vi "Console.vi"() -> ()   [LabVIEW 2017]
uses:
  Print Options.ctl
panel:
  out "Console Out":string
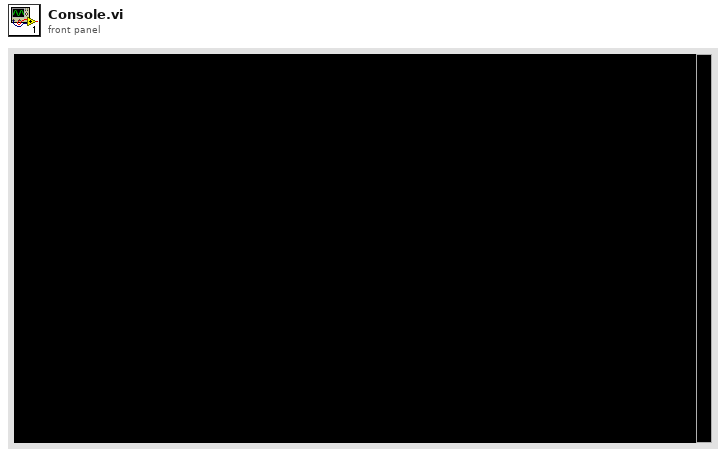
[diagram p1: front panel]
types:
  T1 = typedef "Print Options.ctl" = enum16{"Create", "Get Reference", "Print", "Print Header", "Close"}
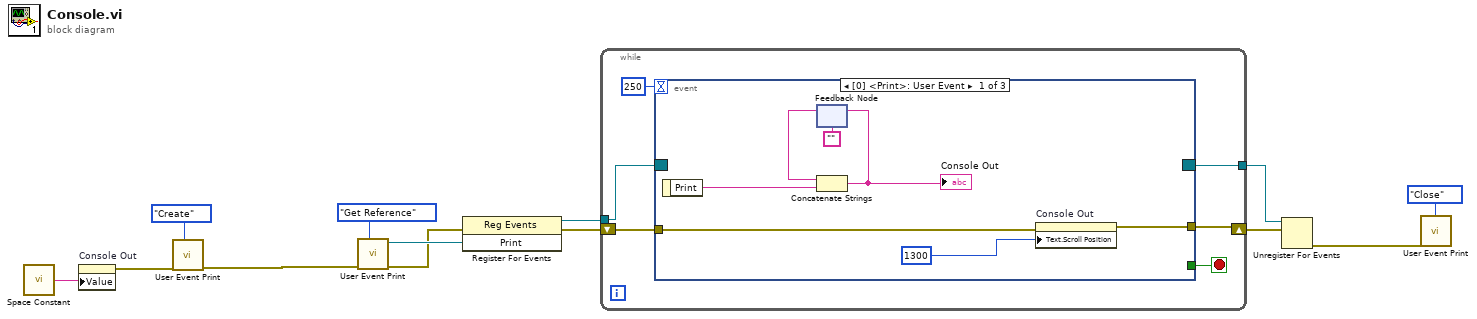
[diagram p0: block diagram]
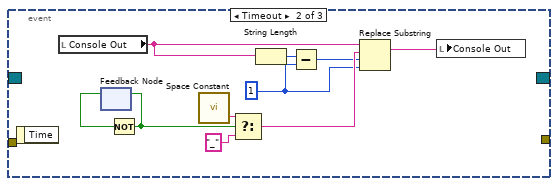
[diagram p2: hidden frame]
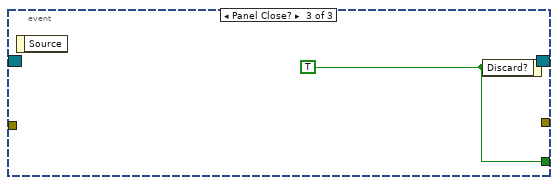
[diagram p3: hidden frame]
diagram:
  n1 = call <vilib>:"Space Constant.vi"() -> ("String"=w4:string)
  n2 = property on="Console Out" class="Str"("Value"=w4) -> (error out=w5:errorcluster)  [unwired: 2 in, 1 out]
  n3 = call "User Event Print.vi"("Options"=Print_Options."Create", "error in (no error)"=w5) -> ("error out"=w7:errorcluster)  [unwired: 8 in, 1 out]
  n4 = call "User Event Print.vi"("Options"=Print_Options."Get Reference", "error in (no error)"=w7) -> ("error out"=w3:errorcluster, "Print"=w6:refnum<user-event>)  [unwired: 8 in]
  n5 = register-events(error in=w3, w6) -> (reference out=w12:refnum<event-registration>, error out=w2:errorcluster)  [unwired: 1 in]
  n6 = while {
    tunnel: w12 -> [w18]
    tunnel: [w17] -> w13
    shift-right: [w14] -> w1
    shift-left: w2 -> [w15]
    stop <- w19 stop-if-true
    n7 = event shown="[0] <Print>: User Event" {
      selector: w18 -> [_ _ _]
      dyn-events: [_ _ _] -> w17
      timeout: 250 -> [_ _ _]
      tunnel: [_ _ w37] -> w19
      tunnel: w15 -> [w21 _ _]
      tunnel: [w20 _ _] -> w14
      event User Event {
        n8 = event-data() -> ("Print"=w26:string)  [unwired: 1 in]
        n9 = feedback #1("") -> (w25:string)
        n10 = Concatenate Strings(w25, w26) -> (w23:string)
        "Console Out" <- w23
        n11 = feedback-in #1(w23) -> ()
        n12 = property on="Console Out" class="Str"(error in=w21, "Text.Scroll Position"=u32 1300) -> (error out=w20:errorcluster)  [unwired: 1 in, 1 out]
      }
      event Timeout {
        w29 = 1 ("length (len. of substring)")
        n13 = event-data() -> ()  [unwired: 1 in, 1 out]
        n14 = local read "Console Out"() -> (w34:string)
        n15 = feedback #2() -> (w36:bool)  [unwired: 1 in]
        n16 = Not(x=w36) -> (.not. x?=w33:bool)
        n17 = feedback-in #2(w33) -> ()
        n18 = call <vilib>:"Space Constant.vi"() -> ("String"=w28:string)
        n19 = Select(t=w28, s=w33, f="_") -> (s? t:f=w32:string)
        n20 = String Length(string=w34) -> (length=w31:i32)
        n21 = Subtract(x=w31, y=w29) -> (x-y=w30:i32)
        n22 = Replace Substring(2:w29, 3:w30, 4:w32, 5:w34) -> (1:w35:string)  [unwired: 1 out]
        n23 = local write "Console Out"(w35) -> ()
      }
      event Panel Close? {
        w37 = TRUE ("Discard?")
        n24 = event-data() -> ()  [unwired: 1 in, 1 out]
        n25 = event-data("Discard?"=w37) -> ()  [unwired: 1 in, 1 out]
      }
    }
  }
  n26 = Unregister For Events(event registration refnum=w13, error in=w1) -> (error out=w11:errorcluster)
  n27 = call "User Event Print.vi"("Options"=Print_Options."Close", "error in (no error)"=w11) -> ()  [unwired: 8 in, 2 out]
